vi "Permanentes.vi"() -> ()   [LabVIEW 2013]
panel:
  in  "Recetas_Selector":cluster{"String":string, "Value":ext}[](array[cluster])
  in  "Programa":T1
  in  "Recetas Allen Bradley":T2(array[cluster]) {"Modbus PowerFlex"."Tmp. pérdida comun." min=0.0 max=60.0 format="%#_g seg."; "Modbus PowerFlex"."Identificador" min=1 max=247; "Modbus PowerFlex"."Formato RS485" items=["RTU 8-N-1", "RTU 8-E-1", "RTU 8-O-1", "RTU 8-N-2", "RTU 8-E-2", "RTU 8-O-2"]; "Modbus PowerFlex"."Acc. pérdida comun." items=["Fallo", "Paro inercia", "Paro", "Nada"]; "Modbus PowerFlex"."Velocidad datos" items=["9600 bps", "2400 bps", "4800 bps", "9600 bps", "19200 bps", "38400 bps"]; "Motor PowerFlex"."T. Desaleceración" format="%#_g seg"; "Motor PowerFlex"."T. Aceleración" format="%#_g seg"; "Motor PowerFlex"."Velocidad nominal" format="%.0f rpm"; "Motor PowerFlex"."Voltaje nominal" format="%.0f V"; "Motor PowerFlex"."Frecuencia nominal" format="%.0f Hz"; "Motor PowerFlex"."Corriente sobrecarga" format="%#_g Amp"; "Motor PowerFlex"."Corriente nominal" format="%#_g Amp"; "Motor PowerFlex"."Polos" min=2 max=40; "I/O PowerFlex"."Relevador" items=["Listo/Fallo"=0, "A frecuencia"=1, "Alimentación"=2, "Sobrefrecuencia"=6, "Sobrecorriente"=7, "Sobretensión"=8, "Modbus"=13]; "I/O PowerFlex"."Entrada 6 (06)" items=["No asignar"=0, "Referencia vel. 2"=1, "Referencia vel. 3"=2, "Fallo auxiliar"=12, "Reset"=13, "Entrada lógica 1"=24, "Entrada lógica 2"=25]; "I/O PowerFlex"."Entrada 5 (05)" items=["No asignar"=0, "Referencia vel. 2"=1, "Referencia vel. 3"=2, "Fallo auxiliar"=12, "Reset"=13, "Entrada lógica 1"=24, "Entrada lógica 2"=25]; "I/O PowerFlex"."Entrada 3 (03)" items=["No asignar"=0, "Referencia vel. 2"=1, "Referencia vel. 3"=2, "Fallo auxiliar"=12, "Reset"=13, "Entrada lógica 1"=24, "Entrada lógica 2"=25, "REV 2 hilos"=50, "DIR 3 hilos"=51]; "I/O PowerFlex"."Entrada 2 (02)" items=["No asignar"=0, "Referencia vel. 2"=1, "Referencia vel. 3"=2, "Fallo auxiliar"=12, "Reset"=13, "Entrada lógica 1"=24, "Entrada lógica 2"=25, "FWD 2 hilos"=48, "RUN 3 hilos"=49]; "Referencias PowerFlex"."Referencia velocidad 2" items=["Potenciómetro"=1, "Teclado"=2, "Modbus"=3, "Analógica (0-10V)"=5, "Analógica (4-20mA)"=6]; "Referencias PowerFlex"."Referencia arranque 2" items=["Teclado"=1, "Terminales"=2, "Modbus"=3]; "Referencias PowerFlex"."Referencia velocidad 1" items=["Potenciómetro"=1, "Teclado"=2, "Modbus"=3, "Analógica (0-10V)"=5, "Analógica (4-20mA)"=6]; "Referencias PowerFlex"."Referencia arranque 1" items=["Teclado"=1, "Terminales"=2, "Modbus"=3]}
  in  "Puerto COM":refnum<visa-resource-name>
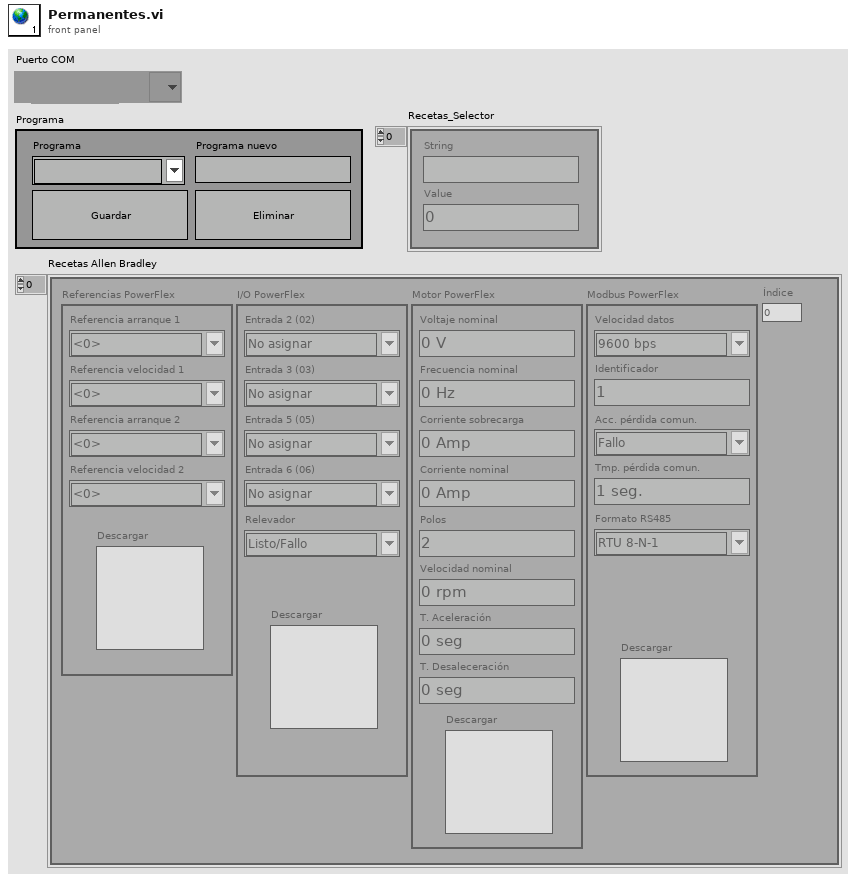
[diagram p1: front panel]
types:
  T1 = cluster{"Guardar":bool, "Eliminar":bool, "Programa":u16, "Programa nuevo":string}
  T2 = cluster{"Referencias PowerFlex":cluster{"Referencia arranque 1":u16, "Referencia velocidad 1":u16, "Referencia arranque 2":u16, "Referencia velocidad 2":u16, "Descargar":bool}, "I/O PowerFlex":cluster{"Entrada 2 (02)":u16, "Entrada 3 (03)":u16, "Entrada 5 (05)":u16, "Entrada 6 (06)":u16, "Relevador":u16, "Descargar":bool}, "Motor PowerFlex":cluster{"Voltaje nominal":u16, "Frecuencia nominal":u16, "Corriente sobrecarga":dbl, "Corriente nominal":dbl, "Polos":u16, "Velocidad nominal":u16, "T. Aceleración":dbl, "T. Desaleceración":dbl, "Descargar":bool}, "Modbus PowerFlex":cluster{"Velocidad datos":u16, "Identificador":u16, "Acc. pérdida comun.":u16, "Tmp. pérdida comun.":dbl, "Formato RS485":u16, "Descargar":bool}, "Índice":u32}[]
diagram:
